vi "Read Class Path.vi"(11 "Message Scripter in":refnum<class "Message Scripter.lvclass">) -> (2 "Class Path":path)   [LabVIEW 2020, in "Message Maker.lvlib" / "Message Scripter.lvclass"]
uses:
  Message Scripter.lvclass
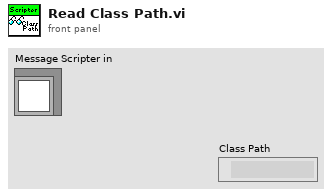
[diagram p1: front panel]
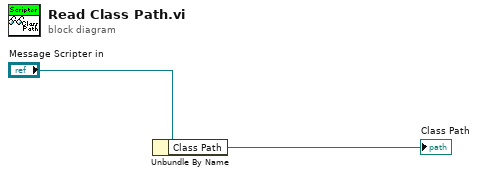
[diagram p0: block diagram]
diagram:
  n1 = Unbundle By Name("Message Scripter in") -> ("Class Path"=→"Class Path":path)
